vi "Image rotate (from file).vi"(0 "Image file path":path=path "C:/Users/Paul Nathan/Desktop/Turntable test 3/Datum_Turntable_2.jpg", 5 "Rotated image file path":path=path "C:/Users/Paul Nathan/Desktop/Turntable test 3/Datum_Turntable_2_X.jpg", 7 "Rotation angle, ccw+ (deg)":dbl, 9 "Quality":u32=750 max=1000, 11 "Error in":errorcluster) -> (15 "Error Out":errorcluster)   [LabVIEW 2015]
panel:
  out "Image out":T1(plugin-control)
  # "PN 18/03/2016"
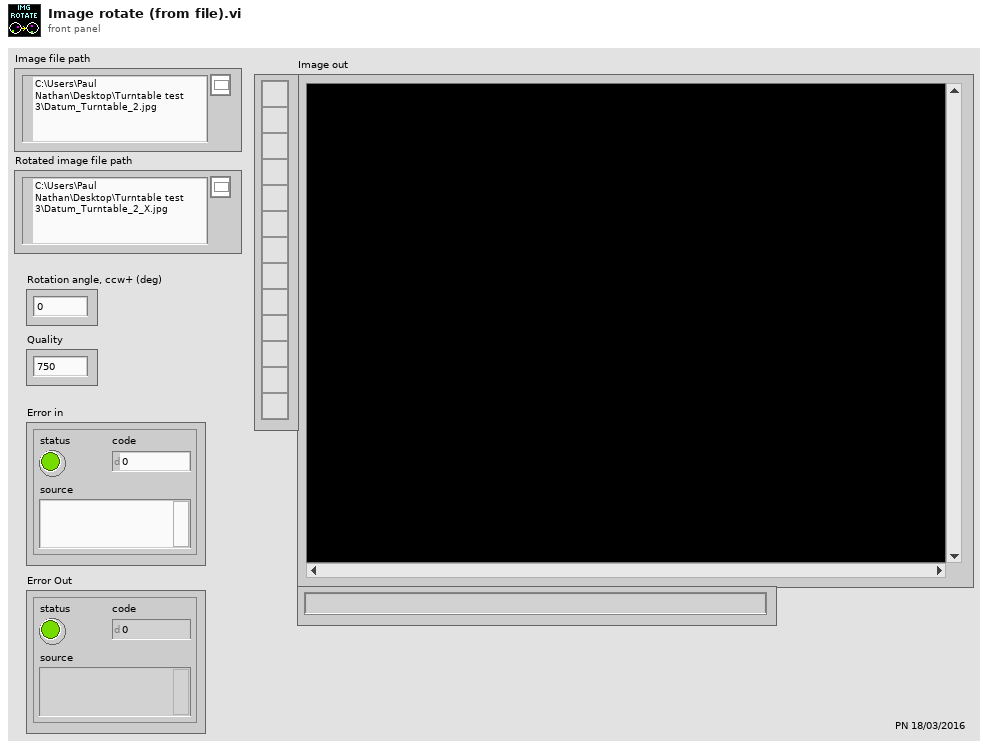
[diagram p1: front panel]
types:
  T1 = typedef "IMAQ Image.ctl" = refnum<image>
  T2 = typedef "Image Type" = u32
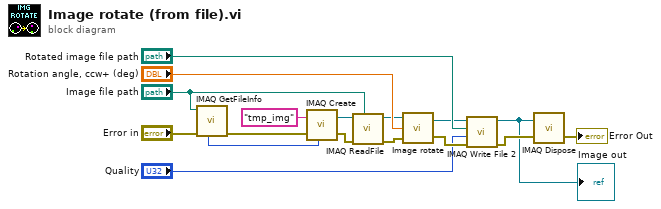
[diagram p0: block diagram]
diagram:
  n1 = call "IMAQ GetFileInfo"("error in (no error)"="Error in", "File Path"="Image file path") -> ("error out"=w14:errorcluster, "Image Type"=w13:T2)  [unwired: 3 in, 5 out]
  n2 = call "IMAQ Create"("Image Name"="tmp_img", "Image Type"=w13, "error in (no error)"=w14) -> ("New Image"=w16:T1, "error out"=w15:errorcluster)  [unwired: 2 in]
  n3 = call "IMAQ ReadFile"("File Path"="Image file path", "error in (no error)"=w15, "Image"=w16) -> ("error out"=w7:errorcluster, "Image Out"=w4:T1)  [unwired: 4 in, 3 out]
  n4 = call "Image rotate.vi"("Error in"=w7, "Rotation angle, ccw+ (deg)"="Rotation angle, ccw+ (deg)", "Image in"=w4) -> ("Error Out"=w6:errorcluster, "Image Out"=w3:T1)
  n5 = call-poly "IMAQ Write File 2"("error in (no error)"=w6, "Image Quality"="Quality", "File Path"="Rotated image file path", "Image"=w3) -> ("error out"=w12:errorcluster, "Image Out (duplicate)"=w8:T1)  [unwired: 6 in]
  "Image out" <- w8
  n6 = call "IMAQ Dispose"("Image"=w8, "error in (no error)"=w12) -> ("error out"=→"Error Out":errorcluster)  [unwired: 4 in]
